vi "Factory Create.vi"(8 "Error In":errorcluster, 10 "IConfigure":refnum<class "IConfigure.lvclass">, 11 "reference in":refnum<class "Instrument Base.lvclass">) -> (0 "Error Out":errorcluster, 3 "reference out":refnum<class "Instrument Base.lvclass">)   [LabVIEW 2023, in "HAL GOOP4.lvlib" / "Instrument Base.lvclass"]
uses:
  Instrument Base.lvclass
  Instrument Base.lvclass/Instrument Base.ctl
  Interfaces/IConfigure/IConfigure.lvclass
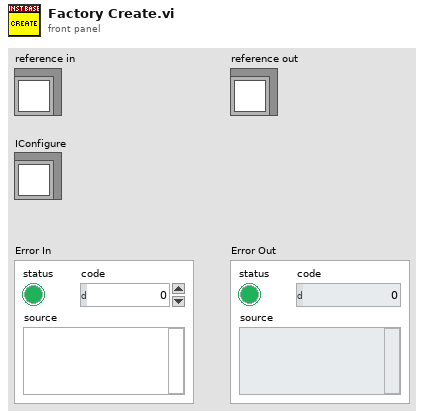
[diagram p1: front panel]
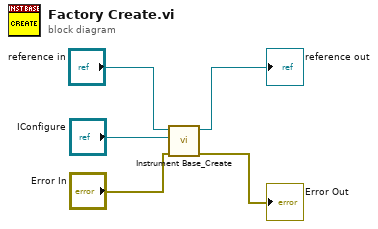
[diagram p0: block diagram]
diagram:
  n1 = call "Instrument Base_Create.vi"("Error In"="Error In", "IConfigure.lvclass"="IConfigure", "reference in"="reference in") -> ("Error Out"=→"Error Out":errorcluster, "reference out"=→"reference out":refnum<class "Instrument Base.lvclass">)  [unwired: 7 in]
